vi "Obtain Broadcast Events.vi"(8 "error in":errorcluster, 10 "Create New? (F)":bool) -> (0 "error out":errorcluster, 2 "Sequence Engine Broadcast Events":T1)   [LabVIEW 2021, in "Sequence Engine.lvlib"]
doc: "This VI Obtains/Creates the Broadcast events that will be used for other modules to register to receive messages from the module that owns this VI.\n\n<b>NOTE</b>: The contents of this VI are automatically generated and modified by the <b>Tools > DQMH Consortium > DQMH</b> utilities. Consider using those utilities instead of making your own modifications to this VI.\n_____\nBased on DQMH Dev Tools: Project Template 7.1.1.1528."
uses:
  Sequence Engine.lvlib
  Broadcast Events--cluster.ctl
  Did Init Argument--cluster.ctl
  Status Updated Argument--cluster.ctl
  Error Reported Argument--cluster.ctl
  Stop Argument--cluster.ctl
  Get Module Execution Status Argument--cluster.ctl
  New Test Result Argument--cluster.ctl
  Classes/Test Result/Result Data.ctl
  Classes/Test Result/Test Status.ctl
  Testing Started Argument--cluster.ctl
  Testing Completed Argument--cluster.ctl
  Retried Count Argument--cluster.ctl
  DUT Info Argument--cluster.ctl
  DUT Info.ctl
  Classes/Test Result/Test Result.lvclass
  Stop Testing Argument--cluster.ctl
panel:
  # "NOTE: The contents of this VI are automatically generated and modified by the Tools > DQMH Consortium > DQMH utilities. Consider using those utilities instead of making your own modifications to this VI."
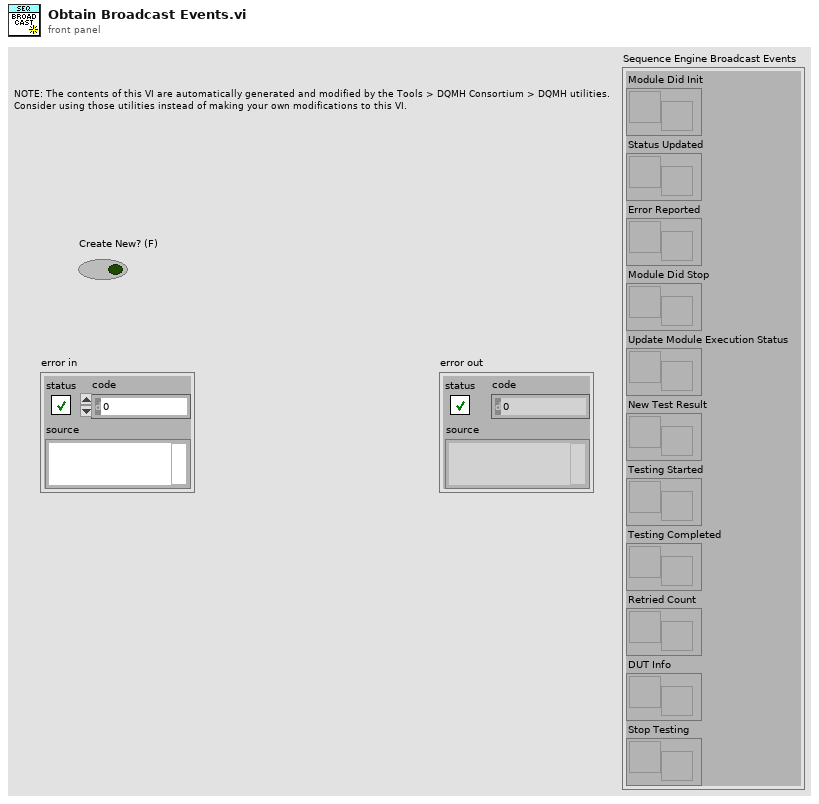
[diagram p1: front panel]
types:
  T1 = typedef "Sequence Engine.lvlib/Broadcast Events--cluster.ctl" = cluster{"Module Did Init":refnum<user-event>, "Status Updated":refnum<user-event>, "Error Reported":refnum<user-event>, "Module Did Stop":refnum<user-event>, "Update Module Execution Status":refnum<user-event>, "New Test Result":refnum<user-event>, "Testing Started":refnum<user-event>, "Testing Completed":refnum<user-event>, "Retried Count":refnum<user-event>, "DUT Info":refnum<user-event>, "Stop Testing":refnum<user-event>}
  T2 = typedef "Sequence Engine.lvlib/Stop Testing Argument--cluster.ctl" = cluster{"Boolean":bool}
  T3 = typedef "Sequence Engine.lvlib/DUT Info Argument--cluster.ctl" = cluster{"DUT Info":T4}
  T4 = typedef "Sequence Engine.lvlib/DUT Info.ctl" = cluster{"Serial Number":string, "Model Number":string}
  T5 = typedef "Sequence Engine.lvlib/Retried Count Argument--cluster.ctl" = cluster{"Retried Count":u16}
  T6 = typedef "Sequence Engine.lvlib/Testing Completed Argument--cluster.ctl" = cluster{"Boolean":bool}
  T7 = typedef "Sequence Engine.lvlib/Testing Started Argument--cluster.ctl" = cluster{"Boolean":bool}
  T8 = typedef "Sequence Engine.lvlib/New Test Result Argument--cluster.ctl" = cluster{"Result Data":T9}
  T9 = typedef "Sequence Engine.lvlib/Test Result.lvclass/Result Data.ctl" = cluster{"Test ID":u32, "Test Name":string, "Sub Test Name":string, "Test Status":T10, "Start Time":timestamp, "End Time":timestamp, "Duration (s)":dbl, "Expected Values":string, "Measured Values":string, "Remarks":string}
  T10 = typedef "Sequence Engine.lvlib/Test Result.lvclass/Test Status.ctl" = enum16{"Pass", "Fail", "Aborted", "Skipped"}
  T11 = typedef "Sequence Engine.lvlib/Get Module Execution Status Argument--cluster.ctl" = cluster{"Running?":bool}
  T12 = typedef "Sequence Engine.lvlib/Stop Argument--cluster.ctl" = cluster{"Origin":string, "Exit via Stop Module Req?":bool, "Wait for Module to stop?":bool}
  T13 = typedef "Sequence Engine.lvlib/Error Reported Argument--cluster.ctl" = cluster{"Error":errorcluster, "Additional Information":string, "Module Name":string}
  T14 = typedef "Sequence Engine.lvlib/Status Updated Argument--cluster.ctl" = cluster{"Status":string}
  T15 = typedef "Sequence Engine.lvlib/Did Init Argument--cluster.ctl" = cluster{"Init?":bool, "Info":string}
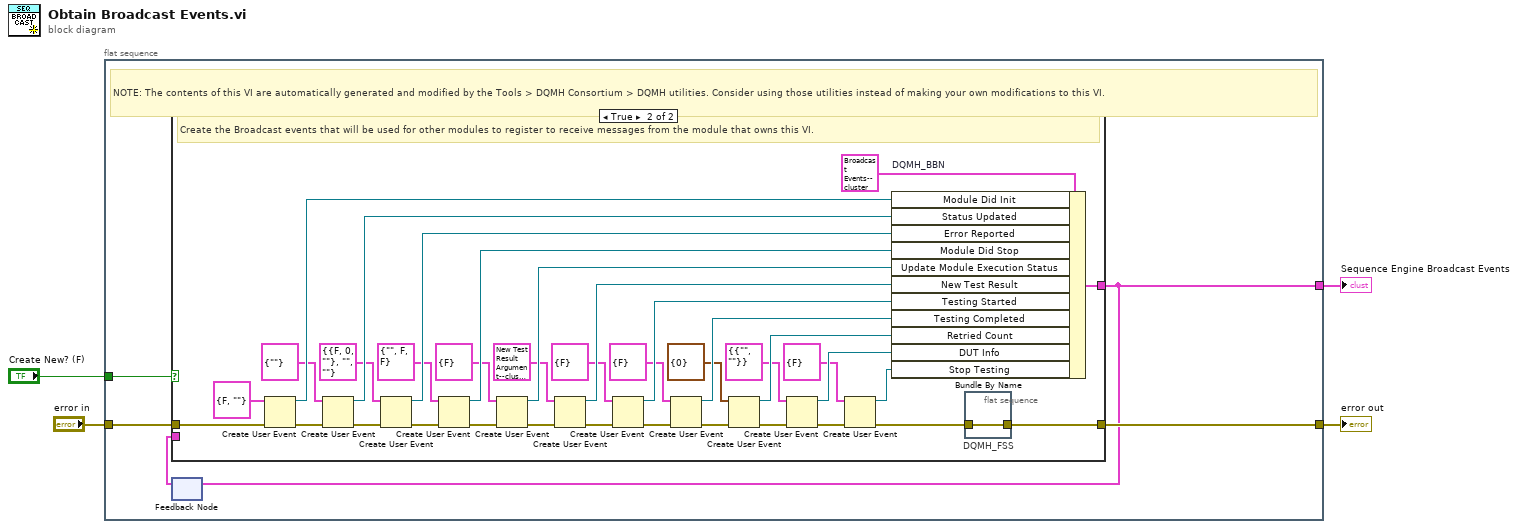
[diagram p0: block diagram]
diagram:
  n1 = flat-sequence {
    tunnel: [w9] -> w4
    tunnel: "error in" -> [w8]
    tunnel: [w6] -> w1
    tunnel: "Create New? (F)" -> [w5]
    frame #0 {
      # "NOTE: The contents of this VI are automatically generated and modified by the Tools > DQMH Consortium > DQMH utilities. Consider using those utilities instead of making your own modifications to this VI."
      n2 = feedback #1() -> (w7:T1)  [unwired: 1 in]
      n3 = case shown="True" w5 {
        tunnel: [w10 w33] -> w9
        tunnel: w8 -> [w10 w48]
        tunnel: [w11 w45] -> w6
        tunnel: w7 -> [w11 _]
        frame False {
          # "Obtain the Broadcast events that were created in a previous call to this VI."
        }
        frame True {
          # "Create the Broadcast events that will be used for other modules to register to receive messages from the module that owns this VI."
          n4 = Create User Event(user event datatype=T15 {"Init?"=FALSE, "Info"=""} ("Did Init Argument"), error in=w48) -> (user event=w46:refnum<user-event>, error out=w43:errorcluster)
          n5 = Create User Event(user event datatype=T14 {"Status"=""} ("Status Updated Argument"), error in=w43) -> (user event=w40:refnum<user-event>, error out=w42:errorcluster)
          n6 = Create User Event(user event datatype=T13 {"Error"={"status"=FALSE, "code"=0, "source"=""}, "Additional Information"="", "Module Name"=""} ("Error Reported Argument"), error in=w42) -> (user event=w37:refnum<user-event>, error out=w39:errorcluster)
          n7 = Create User Event(user event datatype=T12 {"Origin"="", "Exit via Stop Module Req?"=FALSE, "Wait for Module to stop?"=FALSE} ("Stop Argument"), error in=w39) -> (user event=w35:refnum<user-event>, error out=w34:errorcluster)
          n8 = Create User Event(user event datatype=T11 {"Running?"=FALSE} ("Get Module Execution Status Argument"), error in=w34) -> (user event=w31:refnum<user-event>, error out=w32:errorcluster)
          n9 = Create User Event(user event datatype=T8 {"Result Data"={"Test ID"=0, "Test Name"="", "Sub Test Name"="", "Test Status"=enum."Pass", "Start Time"=timestamp(0 s since 1904-01-01), "End Time"=timestamp(0 s since 1904-01-01), "Duration (s)"=0.0, "Expected Values"="", "Measured Values"="", "Remarks"=""}} ("New Test Result Argument"), error in=w32) -> (user event=w28:refnum<user-event>, error out=w29:errorcluster)
          n10 = Create User Event(user event datatype=T7 {"Boolean"=FALSE} ("Testing Started Argument"), error in=w29) -> (user event=w25:refnum<user-event>, error out=w26:errorcluster)
          n11 = Create User Event(user event datatype=T6 {"Boolean"=FALSE} ("Testing Completed Argument"), error in=w26) -> (user event=w22:refnum<user-event>, error out=w23:errorcluster)
          n12 = Create User Event(user event datatype=T5 {"Retried Count"=0} ("Retried Count Argument"), error in=w23) -> (user event=w19:refnum<user-event>, error out=w20:errorcluster)
          n13 = Create User Event(user event datatype=T3 {"DUT Info"={"Serial Number"="", "Model Number"=""}} ("DUT Info Argument"), error in=w20) -> (user event=w16:refnum<user-event>, error out=w17:errorcluster)
          n14 = Create User Event(user event datatype=T2 {"Boolean"=FALSE} ("Stop Testing Argument"), error in=w17) -> (user event=w13:refnum<user-event>, error out=w14:errorcluster)
          n15 = Bundle By Name "DQMH_BBN"(cluster=T1 {"Module Did Init"=refnum, "Status Updated"=refnum, "Error Reported"=refnum, "Module Did Stop"=refnum, "Update Module Execution Status"=refnum, "New Test Result"=refnum, "Testing Started"=refnum, "Testing Completed"=refnum, "Retried Count"=refnum, "DUT Info"=refnum, "Stop Testing"=refnum} ("output cluster"), "Module Did Init"=w46, "Status Updated"=w40, "Error Reported"=w37, "Module Did Stop"=w35, "Update Module Execution Status"=w31, "New Test Result"=w28, "Testing Started"=w25, "Testing Completed"=w22, "Retried Count"=w19, "DUT Info"=w16, "Stop Testing"=w13) -> (w45:T1)
          n16 = flat-sequence "DQMH_FSS" {
            tunnel: w14 -> [w49]
            tunnel: [w49] -> w33
            frame #0 {
            }
          }
        }
      }
      n17 = feedback-in #1(w6) -> ()
    }
  }
  "error out" <- w4
  "Sequence Engine Broadcast Events" <- w1
